vi "4031V6Project.vi"() -> ()   [LabVIEW 2024]
uses:
  <vilib>/Utility/TradDaqScaling.llb/Convert Thermocouple Reading (array).vi
  <vilib>/express/express arith-compare/Formula/XNode/ExpressFormulaBlockNode.xnode
  <vilib>/Utility/file.llb/Write Delimited Spreadsheet (DBL).vi
  <vilib>/Utility/file.llb/Write Delimited Spreadsheet (string).vi
  <vilib>/Analysis/NI_AALBase.lvlib
panel:
  in  "Thermistor Resistance Reading":dbl format="%#_13g"
  out "Cold in":dbl[](graph)
  out "Hot Out":dbl[](graph)
  out "Hot in":dbl[](graph)
  out "Tco SD":dbl
  out "Tci SD":dbl
  out "Tho SD":dbl
  out "Thi SD":dbl
  out "Hot side Delta":dbl format="%#_13g"
  out "Cold Side Delta":dbl format="%#_13g"
  in  "Sampling rate":dbl
  in  "Number of Samples":dbl
  out "Tco Mean":dbl
  out "Tci Mean":dbl
  out "Tho Mean":dbl
  out "Thi Mean":dbl
  out "Cold Out":dbl[](graph)
  in  "?":bool
  # "TEMPERATURE STANDARD DEVIATION"
  # "INPUTS"
  # "MEAN TEMPERATURES"
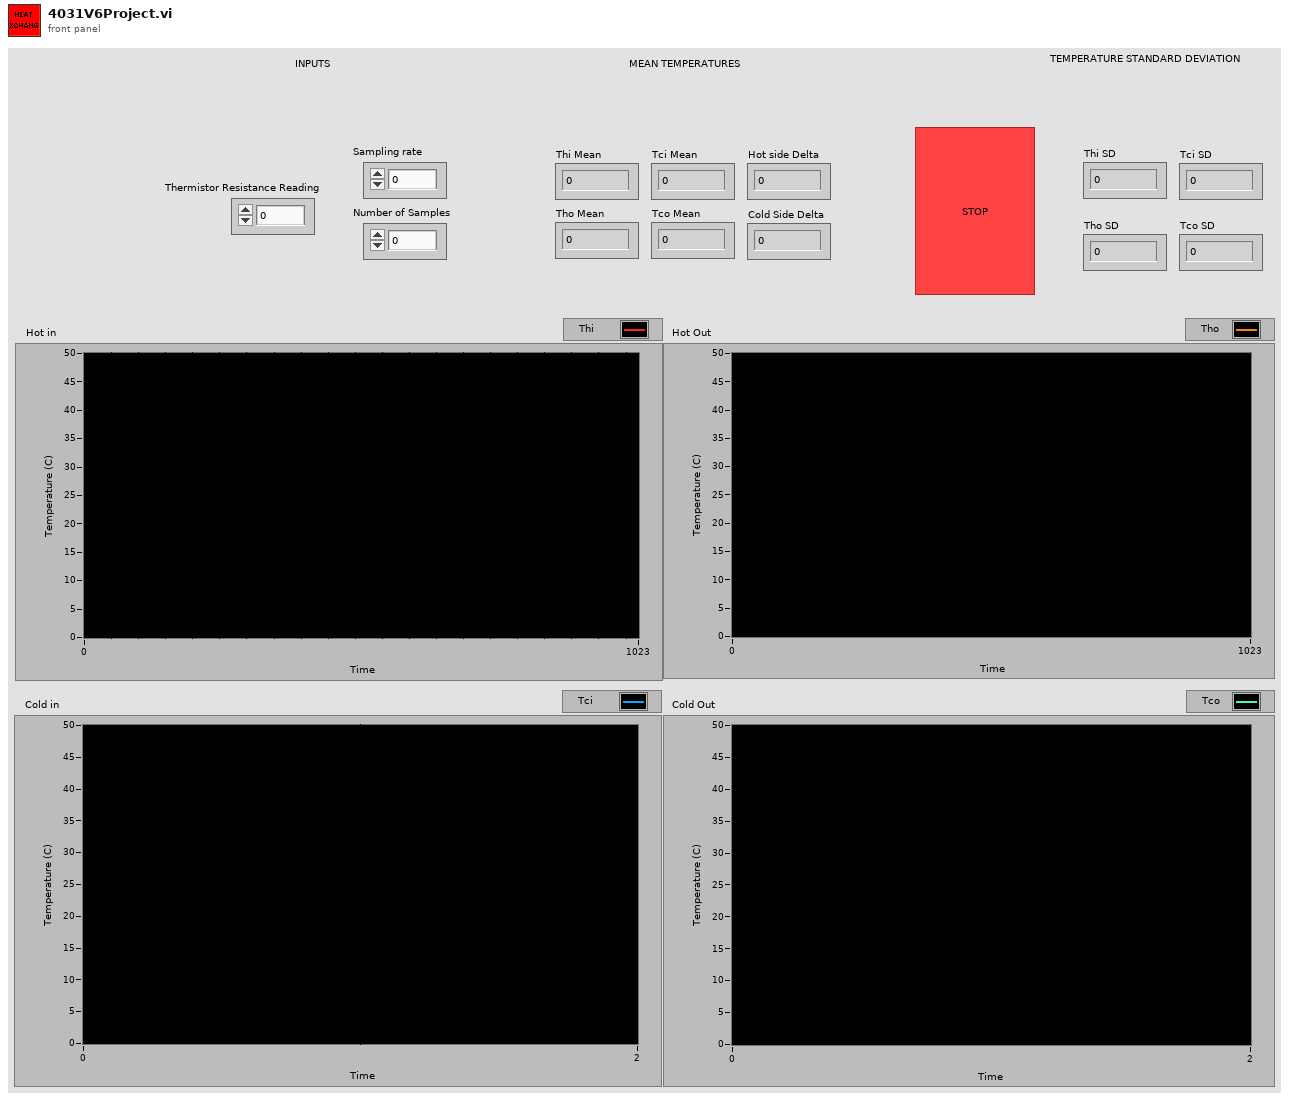
[diagram p1: front panel]
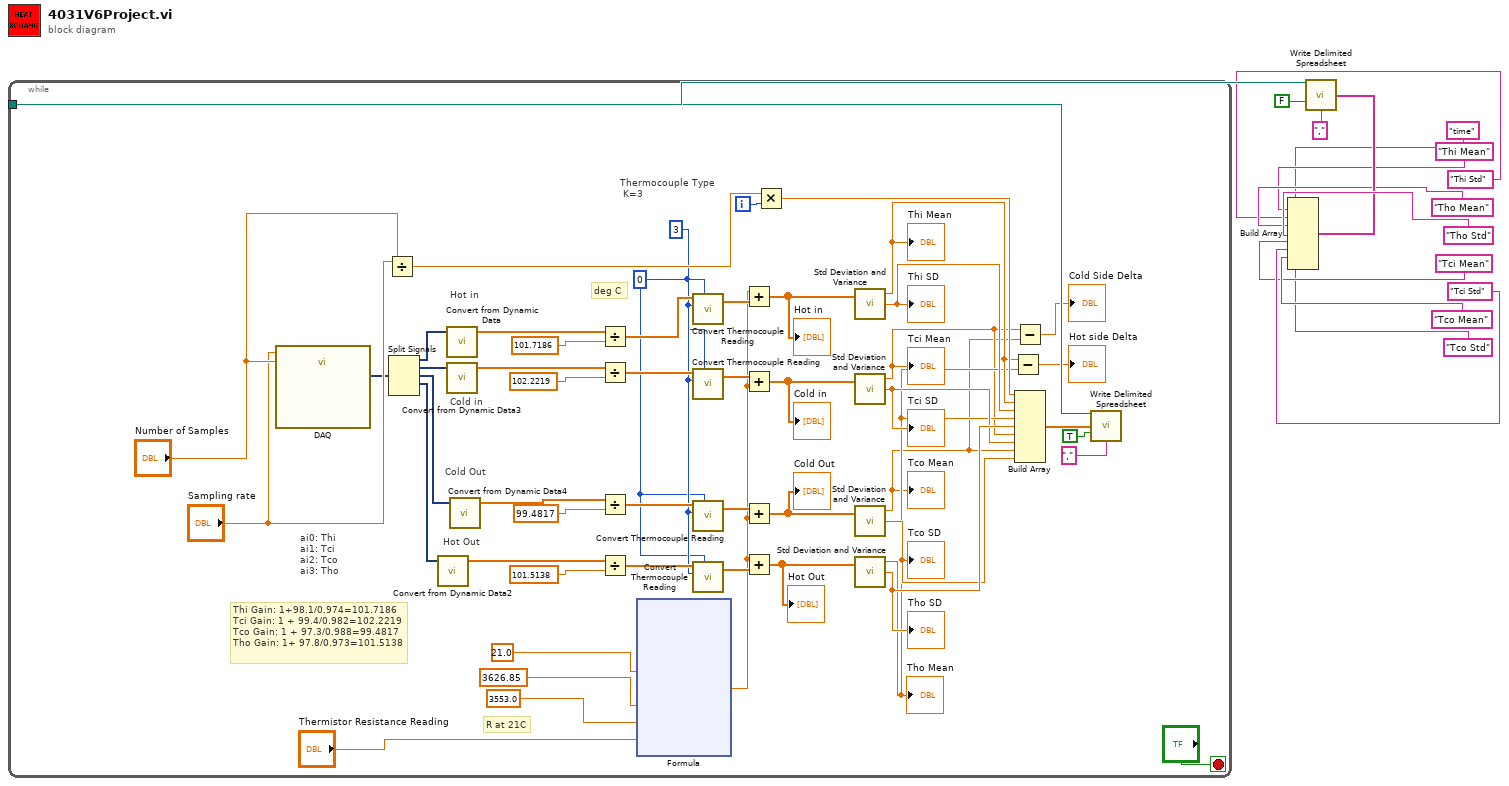
[diagram p0: block diagram]
diagram:
  n1 = Build Array("time", "Thi Mean", "Thi Std", "Tho Mean", "Tho Std", "Tci Mean", "Tci Std", "Tco Mean", "Tco Std") -> (w9:string[])
  n2 = call-poly <vilib>:"Write Delimited Spreadsheet.vi"("1D data"=w9, "append to file? (new file:F)"=FALSE, "delimiter (\\t)"=",") -> ("new file path (Not A Path if cancelled)"=w7:path)  [unwired: 11 in, 1 out]
  n3 = while {
    tunnel: w7 -> [w61]
    i -> [w50]
    stop <- "?" stop-if-true
    w28 = 0
    w29 = 3
    # "Cold in"
    # "R at 21C"
    # "deg C"
    # "Thi Gain: 1+98.1/0.974=101.7186\nTci Gain: 1 + 99.4/0.982=102.2219\nTco Gain: 1 + 97.3/0.988=99.4817\nTho Gain: 1+ 97.8/0.973=101.5138"
    # "ai0: Thi\nai1: Tci\nai2: Tco\nai3: Tho"
    # "Thermocouple Type\n K=3"
    # "Hot Out"
    # "Cold Out"
    # "Hot in"
    n4 = call "DAQ"("rate"="Sampling rate", "number of samples"="Number of Samples") -> ("data"=w35:dynamicdata)  [unwired: 15 in, 2 out]
    n5 = Divide(x="Sampling rate", y="Number of Samples") -> (x/y=w57:dbl)
    n6 = Split Signals(w35) -> (w34:dynamicdata, w33:dynamicdata, w32:dynamicdata, w31:dynamicdata)  [unwired: 5 in, 1 out]
    n7 = call "Convert from Dynamic Data2"("Dynamic Data Type"=w31) -> ("Array"=w55:dbl[])  [unwired: 3 in]
    n8 = call "Convert from Dynamic Data"("Dynamic Data Type"=w34) -> ("Array"=w59:dbl[])  [unwired: 3 in]
    n9 = call "Convert from Dynamic Data3"("Dynamic Data Type"=w33) -> ("Array"=w49:dbl[])  [unwired: 3 in]
    n10 = call "Convert from Dynamic Data4"("Dynamic Data Type"=w32) -> ("Array"=w27:dbl[])  [unwired: 3 in]
    n11 = Divide(x=w59, y=101.7186) -> (x/y=w58:dbl[])
    n12 = Divide(x=w49, y=102.2219) -> (x/y=w30:dbl[])
    n13 = Divide(x=w27, y=99.4817) -> (x/y=w51:dbl[])
    n14 = Divide(x=w55, y=101.5138) -> (x/y=w54:dbl[])
    n15 = xnode ("Formula")("T1"=21.0, "B"=3626.85, "R1"=3553.0, "R2"="Thermistor Resistance Reading") -> ("Result"=w14:dbl)  [unwired: 1 in, 1 out]
    n16 = call-poly <vilib>:"Convert Thermocouple Reading.vi"("Temperature Units (C)"=w28, "ThermocoupleType"=w29, "Voltage Array"=w58) -> ("Temperature Array"=w22:sgl[])  [unwired: 4 in]
    n17 = call-poly <vilib>:"Convert Thermocouple Reading.vi"("Temperature Units (C)"=w28, "ThermocoupleType"=w29, "Voltage Array"=w30) -> ("Temperature Array"=w18:sgl[])  [unwired: 4 in]
    n18 = call-poly <vilib>:"Convert Thermocouple Reading.vi"("Temperature Units (C)"=w28, "ThermocoupleType"=w29, "Voltage Array"=w51) -> ("Temperature Array"=w16:sgl[])  [unwired: 4 in]
    n19 = call-poly <vilib>:"Convert Thermocouple Reading.vi"("Temperature Units (C)"=w28, "ThermocoupleType"=w29, "Voltage Array"=w54) -> ("Temperature Array"=w20:sgl[])  [unwired: 4 in]
    n20 = Add(x=w14, y=w22) -> (x+y=w21:dbl[])
    "Hot in" <- w21
    n21 = Add(x=w18, y=w14) -> (x+y=w17:dbl[])
    "Cold in" <- w17
    n22 = Add(x=w16, y=w14) -> (x+y=w15:dbl[])
    "Cold Out" <- w15
    n23 = Add(x=w14, y=w20) -> (x+y=w19:dbl[])
    "Hot Out" <- w19
    n24 = Multiply(x=w57, y=w50) -> (x*y=w47:dbl)
    n25 = call <vilib>:"Std Deviation and Variance.vi"("X"=w21) -> ("mean"=w39:dbl, "standard deviation"=w48:dbl)  [unwired: 1 in, 1 out]
    "Thi Mean" <- w39
    "Thi SD" <- w48
    n26 = call <vilib>:"Std Deviation and Variance.vi"("X"=w17) -> ("mean"=w37:dbl, "standard deviation"=w45:dbl)  [unwired: 1 in, 1 out]
    "Tci Mean" <- w37
    "Tci SD" <- w45
    n27 = call <vilib>:"Std Deviation and Variance.vi"("X"=w15) -> ("mean"=w36:dbl, "standard deviation"=w44:dbl)  [unwired: 1 in, 1 out]
    "Tco Mean" <- w36
    "Tco SD" <- w44
    n28 = call <vilib>:"Std Deviation and Variance.vi"("X"=w19) -> ("mean"=w38:dbl, "standard deviation"=w46:dbl)  [unwired: 1 in, 1 out]
    "Tho Mean" <- w38
    "Tho SD" <- w46
    n29 = Subtract(x=w39, y=w38) -> (x-y=→"Hot side Delta":dbl)
    n30 = Subtract(x=w37, y=w36) -> (x-y=→"Cold Side Delta":dbl)
    n31 = Build Array(w47, w39, w48, w38, w46, w37, w45, w36, w44) -> (w63:dbl[])
    n32 = call-poly <vilib>:"Write Delimited Spreadsheet.vi"("file path (dialog if empty)"=w61, "1D data"=w63, "append to file? (new file:F)"=TRUE, "delimiter (\\t)"=",") -> ()  [unwired: 10 in, 2 out]
  }
